vi "Manual Error Handling.vi"() -> ()   [LabVIEW 2020]
uses:
  <vilib>/DAQmx/read.llb/DAQmx Read (Analog 1D DBL 1Chan NSamp).vi
  <vilib>/DAQmx/create/channels.llb/DAQmx Create Channel (AI-Acceleration-Accelerometer).vi
  <vilib>/DAQmx/configure/timing.llb/DAQmx Timing (Sample Clock).vi
  <vilib>/DAQmx/miscellaneous.llb/DAQmx Fill In Error Info.vi
panel:
  out "error out":errorcluster
  out "Acceleration Data - Graph":dbl[](graph)
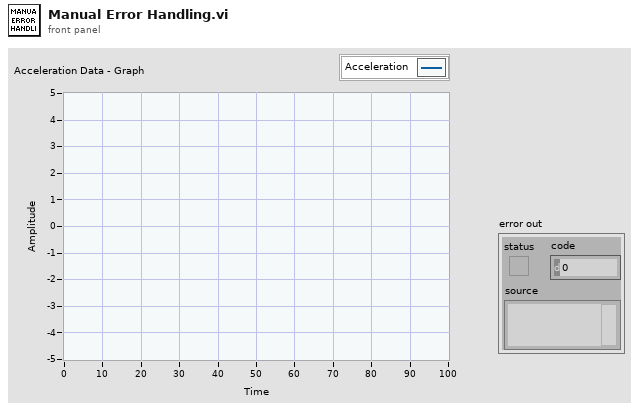
[diagram p1: front panel]
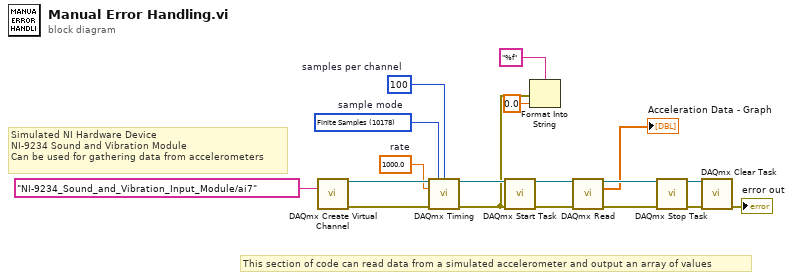
[diagram p0: block diagram]
diagram:
  w10 = 1000.0  # rate
  w11 = 100  # samples per channel
  w12 = 10178 items=["Finite Samples"=10178, "Continuous Samples"=10123, "Hardware Timed Single Point"=12522]  # sample mode
  # "This section of code can read data from a simulated accelerometer and output an array of values"
  # "Simulated NI Hardware Device\nNI-9234 Sound and Vibration Module\nCan be used for gathering data from accelerometers"
  n1 = call-poly <vilib>:"DAQmx Create Virtual Channel.vi"("physical channels"=tag "NI-9234_Sound_and_Vibration_Input_Module/ai7") -> ("task out"=w14:refnum<k21>, "error out"=w8:errorcluster)  [unwired: 13 in]
  n2 = call-poly <vilib>:"DAQmx Timing.vi"("task/channels in"=w14, "sample mode"=w12, "samples per channel"=w11, "rate"=w10, "error in"=w8) -> ("task out"=w13:refnum<k21>, "error out"=w3:errorcluster)  [unwired: 9 in]
  n3 = call <vilib>:"DAQmx Start Task.vi"("task/channels in"=w13, "error in"=w3) -> ("task out"=w18:refnum<k21>, "error out"=w7:errorcluster)  [unwired: 12 in]
  n4 = Format Into String(format string="%f", error in=w3, 0.0 ("input 1")) -> ()  [unwired: 1 in, 2 out]
  n5 = call-poly <vilib>:"DAQmx Read.vi"("task/channels in"=w18, "error in"=w7) -> ("task out"=w16:refnum<k21>, "data"=→"Acceleration Data - Graph":dbl[], "error out"=w6:errorcluster)  [unwired: 11 in]
  n6 = call <vilib>:"DAQmx Stop Task.vi"("task/channels in"=w16, "error in"=w6) -> ("task out"=w17:refnum<k21>, "error out"=w5:errorcluster)  [unwired: 12 in]
  n7 = call <vilib>:"DAQmx Clear Task.vi"("task in"=w17, "error in"=w5) -> ("error out"=→"error out":errorcluster)  [unwired: 13 in]
